vi "Next move 2.vi"(9 "Elevator states in":T1[](array[typedef])=[{"Elevator"={"Up Button"=FALSE, "Current floor"=1, "Down Button"=FALSE, "Car"={"Blank Button"=FALSE, "Blank Button 2"=FALSE, "Blank Button 3"=FALSE, "Blank Button 4"=FALSE, "Blank Button 5"=FALSE, "Blank Button 6"=FALSE, "Blank Button 7"=FALSE, "Blank Button 8"=FALSE, "Blank Button 9"=FALSE, "Blank Button 10"=FALSE, "Blank Button 11"=FALSE, "Blank Button 12"=FALSE, "Blank Button 13"=FALSE, "Blank Button 14"=FALSE, "Blank Button 15"=FALSE, "Blank Button 16"=FALSE, "Blank Button 17"=FALSE, "Blank Button 18"=FALSE, "Blank Button 19"=FALSE, "Blank Button 20"=FALSE}, "Close door"=FALSE}, "Destinations"=[], "Idle floor"=1, "Max floor"=7, "Min floor"=1, "Next floor"=0, "Move started"=timestamp(0 s since 1904-01-01), "Idle move"=FALSE}, {"Elevator"={"Up Button"=FALSE, "Current floor"=8, "Down Button"=FALSE, "Car"={"Blank Button"=FALSE, "Blank Button 2"=FALSE, "Blank Button 3"=FALSE, "Blank Button 4"=FALSE, "Blank Button 5"=FALSE, "Blank Button 6"=FALSE, "Blank Button 7"=FALSE, "Blank Button 8"=FALSE, "Blank Button 9"=FALSE, "Blank Button 10"=FALSE, "Blank Button 11"=FALSE, "Blank Button 12"=FALSE, "Blank Button 13"=FALSE, "Blank Button 14"=FALSE, "Blank Button 15"=FALSE, "Blank Button 16"=FALSE, "Blank Button 17"=FALSE, "Blank Button 18"=FALSE, "Blank Button 19"=FALSE, "Blank Button 20"=FALSE}, "Close door"=FALSE}, "Destinations"=[], "Idle floor"=8, "Max floor"=14, "Min floor"=8, "Next floor"=0, "Move started"=timestamp(0 s since 1904-01-01), "Idle move"=FALSE}, {"Elevator"={"Up Button"=FALSE, "Current floor"=1, "Down Button"=FALSE, "Car"={"Blank Button"=FALSE, "Blank Button 2"=FALSE, "Blank Button 3"=FALSE, "Blank Button 4"=FALSE, "Blank Button 5"=FALSE, "Blank Button 6"=FALSE, "Blank Button 7"=FALSE, "Blank Button 8"=FALSE, "Blank Button 9"=FALSE, "Blank Button 10"=FALSE, "Blank Button 11"=FALSE, "Blank Button 12"=FALSE, "Blank Button 13"=FALSE, "Blank Button 14"=FALSE, "Blank Button 15"=FALSE, "Blank Button 16"=FALSE, "Blank Button 17"=FALSE, "Blank Button 18"=FALSE, "Blank Button 19"=FALSE, "Blank Button 20"=FALSE}, "Close door"=FALSE}, "Destinations"=[], "Idle floor"=1, "Max floor"=14, "Min floor"=1, "Next floor"=0, "Move started"=timestamp(0 s since 1904-01-01), "Idle move"=FALSE}, {"Elevator"={"Up Button"=FALSE, "Current floor"=14, "Down Button"=FALSE, "Car"={"Blank Button"=FALSE, "Blank Button 2"=FALSE, "Blank Button 3"=FALSE, "Blank Button 4"=FALSE, "Blank Button 5"=FALSE, "Blank Button 6"=FALSE, "Blank Button 7"=FALSE, "Blank Button 8"=FALSE, "Blank Button 9"=FALSE, "Blank Button 10"=FALSE, "Blank Button 11"=FALSE, "Blank Button 12"=FALSE, "Blank Button 13"=FALSE, "Blank Button 14"=FALSE, "Blank Button 15"=FALSE, "Blank Button 16"=FALSE, "Blank Button 17"=FALSE, "Blank Button 18"=FALSE, "Blank Button 19"=FALSE, "Blank Button 20"=FALSE}, "Close door"=FALSE}, "Destinations"=[], "Idle floor"=14, "Max floor"=20, "Min floor"=6, "Next floor"=0, "Move started"=timestamp(0 s since 1904-01-01), "Idle move"=FALSE}]) -> (1 "Elevator states out":T1[](array[typedef])=[{"Elevator"={"Up Button"=FALSE, "Current floor"=1, "Down Button"=FALSE, "Car"={"Blank Button"=FALSE, "Blank Button 2"=FALSE, "Blank Button 3"=FALSE, "Blank Button 4"=FALSE, "Blank Button 5"=FALSE, "Blank Button 6"=FALSE, "Blank Button 7"=FALSE, "Blank Button 8"=FALSE, "Blank Button 9"=FALSE, "Blank Button 10"=FALSE, "Blank Button 11"=FALSE, "Blank Button 12"=FALSE, "Blank Button 13"=FALSE, "Blank Button 14"=FALSE, "Blank Button 15"=FALSE, "Blank Button 16"=FALSE, "Blank Button 17"=FALSE, "Blank Button 18"=FALSE, "Blank Button 19"=FALSE, "Blank Button 20"=FALSE}, "Close door"=FALSE}, "Destinations"=[], "Idle floor"=1, "Max floor"=7, "Min floor"=1, "Next floor"=0, "Move started"=timestamp(0 s since 1904-01-01), "Idle move"=FALSE}, {"Elevator"={"Up Button"=FALSE, "Current floor"=8, "Down Button"=FALSE, "Car"={"Blank Button"=FALSE, "Blank Button 2"=FALSE, "Blank Button 3"=FALSE, "Blank Button 4"=FALSE, "Blank Button 5"=FALSE, "Blank Button 6"=FALSE, "Blank Button 7"=FALSE, "Blank Button 8"=FALSE, "Blank Button 9"=FALSE, "Blank Button 10"=FALSE, "Blank Button 11"=FALSE, "Blank Button 12"=FALSE, "Blank Button 13"=FALSE, "Blank Button 14"=FALSE, "Blank Button 15"=FALSE, "Blank Button 16"=FALSE, "Blank Button 17"=FALSE, "Blank Button 18"=FALSE, "Blank Button 19"=FALSE, "Blank Button 20"=FALSE}, "Close door"=FALSE}, "Destinations"=[], "Idle floor"=8, "Max floor"=14, "Min floor"=8, "Next floor"=0, "Move started"=timestamp(0 s since 1904-01-01), "Idle move"=FALSE}, {"Elevator"={"Up Button"=FALSE, "Current floor"=1, "Down Button"=FALSE, "Car"={"Blank Button"=FALSE, "Blank Button 2"=FALSE, "Blank Button 3"=FALSE, "Blank Button 4"=FALSE, "Blank Button 5"=FALSE, "Blank Button 6"=FALSE, "Blank Button 7"=FALSE, "Blank Button 8"=FALSE, "Blank Button 9"=FALSE, "Blank Button 10"=FALSE, "Blank Button 11"=FALSE, "Blank Button 12"=FALSE, "Blank Button 13"=FALSE, "Blank Button 14"=FALSE, "Blank Button 15"=FALSE, "Blank Button 16"=FALSE, "Blank Button 17"=FALSE, "Blank Button 18"=FALSE, "Blank Button 19"=FALSE, "Blank Button 20"=FALSE}, "Close door"=FALSE}, "Destinations"=[], "Idle floor"=1, "Max floor"=14, "Min floor"=1, "Next floor"=0, "Move started"=timestamp(0 s since 1904-01-01), "Idle move"=FALSE}, {"Elevator"={"Up Button"=FALSE, "Current floor"=14, "Down Button"=FALSE, "Car"={"Blank Button"=FALSE, "Blank Button 2"=FALSE, "Blank Button 3"=FALSE, "Blank Button 4"=FALSE, "Blank Button 5"=FALSE, "Blank Button 6"=FALSE, "Blank Button 7"=FALSE, "Blank Button 8"=FALSE, "Blank Button 9"=FALSE, "Blank Button 10"=FALSE, "Blank Button 11"=FALSE, "Blank Button 12"=FALSE, "Blank Button 13"=FALSE, "Blank Button 14"=FALSE, "Blank Button 15"=FALSE, "Blank Button 16"=FALSE, "Blank Button 17"=FALSE, "Blank Button 18"=FALSE, "Blank Button 19"=FALSE, "Blank Button 20"=FALSE}, "Close door"=FALSE}, "Destinations"=[], "Idle floor"=14, "Max floor"=20, "Min floor"=6, "Next floor"=0, "Move started"=timestamp(0 s since 1904-01-01), "Idle move"=FALSE}], 2 "Served floors":u16[](array[numeric]), 5 "Served car":bool[](array[boolean]))   [LabVIEW 2019]
uses:
  Type defs/Elevator states.ctl
  Type defs/Elevator position.ctl
  Type defs/Car buttons.ctl
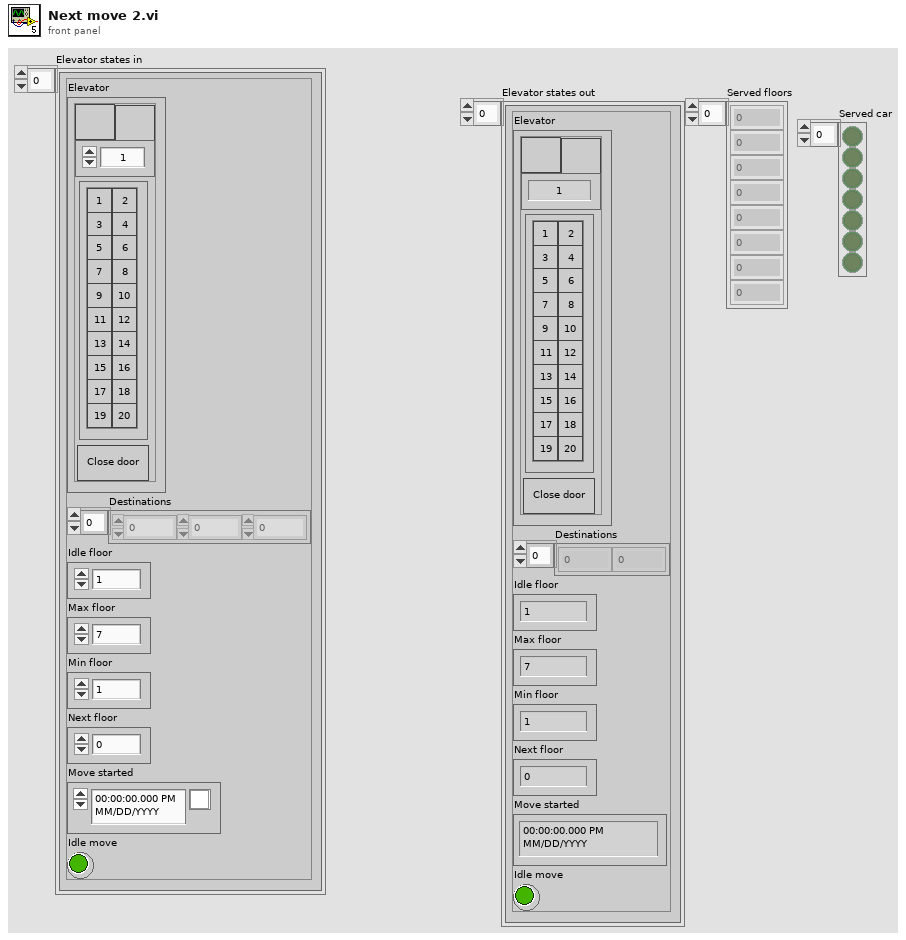
[diagram p1: front panel]
types:
  T1 = typedef "Elevator states.ctl" = cluster{"Elevator":T2, "Destinations":i32[], "Idle floor":u16, "Max floor":u16, "Min floor":u16, "Next floor":u16, "Move started":timestamp, "Idle move":bool}
  T2 = typedef "Elevator position.ctl" = cluster{"Up Button":bool, "Current floor":u16, "Down Button":bool, "Car":T3, "Close door":bool}
  T3 = typedef "Car buttons.ctl" = cluster{"Blank Button":bool, "Blank Button 2":bool, "Blank Button 3":bool, "Blank Button 4":bool, "Blank Button 5":bool, "Blank Button 6":bool, "Blank Button 7":bool, "Blank Button 8":bool, "Blank Button 9":bool, "Blank Button 10":bool, "Blank Button 11":bool, "Blank Button 12":bool, "Blank Button 13":bool, "Blank Button 14":bool, "Blank Button 15":bool, "Blank Button 16":bool, "Blank Button 17":bool, "Blank Button 18":bool, "Blank Button 19":bool, "Blank Button 20":bool}
  T4 = cluster{"Car[0]":bool, "Car[1]":bool, "Car[2]":bool, "Car[3]":bool, "Car[4]":bool, "Car[5]":bool, "Car[6]":bool, "Car[7]":bool, "Car[8]":bool, "Car[9]":bool, "Car[10]":bool, "Car[11]":bool, "Car[12]":bool, "Car[13]":bool, "Car[14]":bool, "Car[15]":bool, "Car[16]":bool, "Car[17]":bool, "Car[18]":bool, "Car[19]":bool}
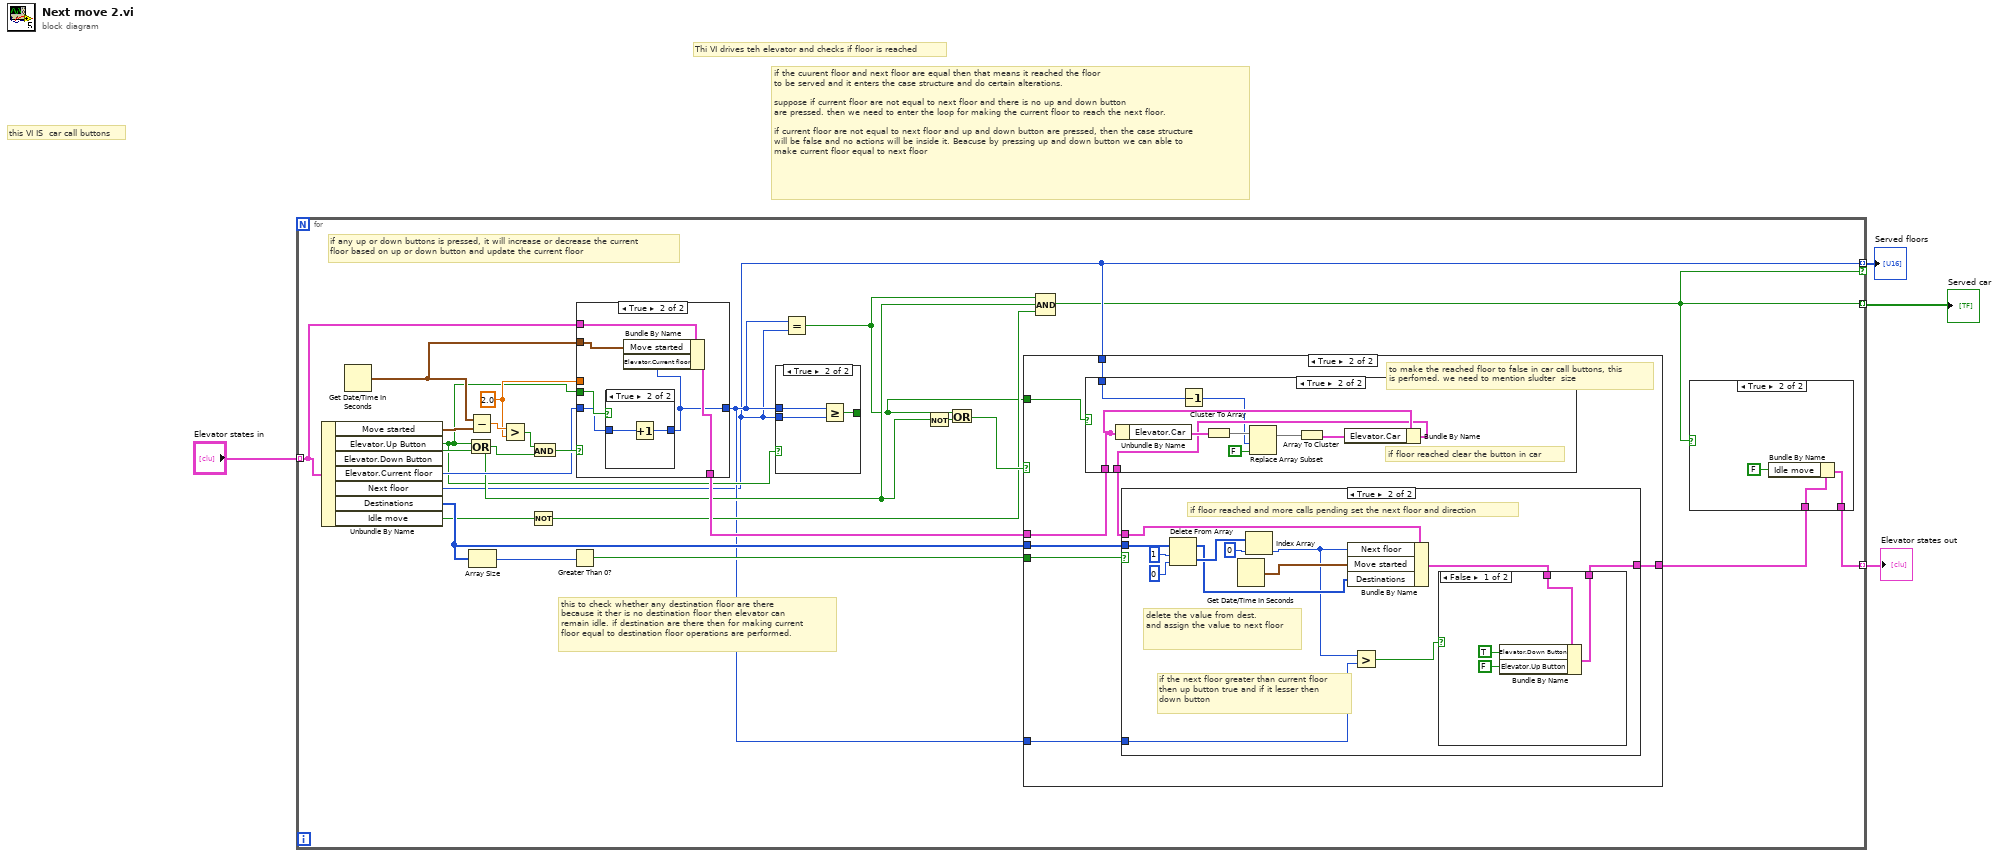
[diagram p0: block diagram]
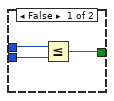
[diagram p2: hidden frame]
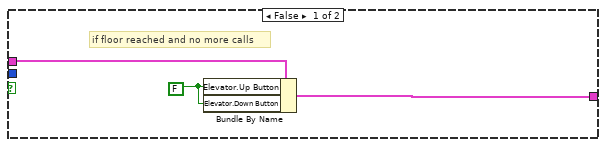
[diagram p5: hidden frame]
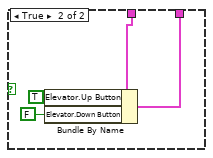
[diagram p6: hidden frame]
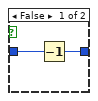
[diagram p9: hidden frame]
diagram:
  # "this VI IS  car call buttons"
  # "if the cuurent floor and next floor are equal then that means it reached the floor\nto be served and it enters the case structure and do certain alterations.\n\nsuppose if current floor are not equal to next floor and there is no up and down button \nare pressed. then we need to enter the loop for making the current floor to reach the next floor.\n\nif current floor are not equal to next floor and up and down button are pressed, then the case structure\nwill be false and no actions will be inside it. Beacuse by pressing up and down button we can able to\nmake current floor equal to next floor"
  # "Thi VI drives teh elevator and checks if floor is reached"
  n1 = for {
    tunnel: "Elevator states in" -> [w19] mode=indexing
    tunnel: [w11] -> w4 mode=indexing
    tunnel: [w7] -> w3 mode=indexing if=w5
    tunnel: [w5] -> w2 mode=indexing
    w24 = 2.0 ("y")
    # "this to check whether any destination floor are there\nbecause it ther is no destination floor then elevator can\nremain idle. if destination are there then for making current\nfloor equal to destination floor operations are performed."
    # "if any up or down buttons is pressed, it will increase or decrease the current\nfloor based on up or down button and update the current floor"
    n2 = Unbundle By Name(w19) -> ("Move started"=w25:timestamp, "Elevator.Up Button"=w9:bool, "Elevator.Down Button"=w29:bool, "Elevator.Current floor"=w18:u16, "Next floor"=w7:u16, "Destinations"=w21:i32[], "Idle move"=w14:bool)
    n3 = Get Date/Time In Seconds() -> (seconds since 1Jan1904=w10:timestamp)
    n4 = Or(x=w9, y=w29) -> (x .or. y?=w15:bool)
    n5 = Subtract(x=w10, y=w25) -> (x-y=w27:dbl)
    n6 = Array Size(array=w21) -> (size(s)=w23:i32)
    n7 = Greater?(x=w27, y=w24) -> (0:w26:bool)
    n8 = Not(x=w14) -> (.not. x?=w13:bool)
    n9 = And(x=w26, y=w15) -> (x .and. y?=w28:bool)
    n10 = Greater Than 0?(x=w23) -> (x > 0?=w22:bool)
    n11 = case shown="True" w28 {
      tunnel: w9 -> [_ w90]
      tunnel: w18 -> [w84 w89]
      tunnel: [w84 w86] -> w8
      tunnel: w19 -> [w83 w88]
      tunnel: w10 -> [_ w85]
      tunnel: w24 -> [_ _]
      tunnel: [w83 w87] -> w20
      frame False {
      }
      frame True {
        n12 = case shown="True" w90 {
          tunnel: w89 -> [w92 w94]
          tunnel: [w91 w93] -> w86
          frame False {
            n13 = Decrement(x=w92) -> (x-1=w91:u16)
          }
          frame True {
            n14 = Increment(x=w94) -> (x+1=w93:u16)
          }
        }
        n15 = Bundle By Name(cluster=w88, "Move started"=w85, "Elevator.Current floor"=w86) -> (w87:T1)
      }
    }
    n16 = case shown="True" w9 {
      tunnel: w8 -> [w32 w35]
      tunnel: w7 -> [w31 w34]
      tunnel: [w30 w33] -> _
      frame False {
        n17 = Less Or Equal?(x=w32, y=w31) -> (x <= y?=w30:bool)
      }
      frame True {
        n18 = Greater Or Equal?(x=w35, y=w34) -> (x >= y?=w33:bool)
      }
    }
    n19 = Equal?(x=w8, y=w7) -> (x = y?=w6:bool)
    n20 = Not(x=w15) -> (.not. x?=w16:bool)
    n21 = Or(x=w6, y=w16) -> (x .or. y?=w17:bool)
    n22 = case shown="True" w17 {
      tunnel: w22 -> [_ w48]
      tunnel: w21 -> [_ w47]
      tunnel: w20 -> [w40 w43]
      tunnel: [w40 w46] -> w12
      tunnel: w8 -> [_ w45]
      tunnel: w7 -> [_ w44]
      tunnel: w6 -> [_ w41]
      frame False {
        # "if floor not reached and elevator is moving"
      }
      frame True {
        # "to make the reached floor to false in car call buttons, this\nis perfomed. we need to mention sludter  size"
        n23 = case shown="True" w41 {
          tunnel: w44 -> [_ w79]
          tunnel: w43 -> [w73 w77]
          tunnel: [w73 w75] -> w42
          frame False {
          }
          frame True {
            # "if floor reached clear the button in car"
            n24 = Unbundle By Name(w77) -> ("Elevator.Car"=w82:T3)
            n25 = Decrement(x=w79) -> (x-1=w74:u16)
            n26 = Cluster To Array(cluster=w82) -> (array=w81:bool[])
            n27 = Replace Array Subset(array=w81, new element=FALSE ("new element/subarray"), index=w74) -> (w78:bool[])
            n28 = Array To Cluster(array=w78) -> (cluster=w76:T4)
            n29 = Bundle By Name(cluster=w77, "Elevator.Car"=w76) -> (w75:T1)
          }
        }
        n30 = case shown="True" w48 {
          tunnel: w47 -> [_ w64]
          tunnel: w42 -> [w51 w59]
          tunnel: [w49 w54] -> w46
          tunnel: w45 -> [_ w52]
          frame False {
            w50 = FALSE ("Elevator.Up Button")
            # "if floor reached and no more calls"
            n31 = Bundle By Name(cluster=w51, "Elevator.Up Button"=w50, "Elevator.Down Button"=w50) -> (w49:T1)
          }
          frame True {
            # "if the next floor greater than current floor\nthen up button true and if it lesser then \ndown button"
            # "delete the value from dest.\nand assign the value to next floor"
            # "if floor reached and more calls pending set the next floor and direction"
            n32 = Delete From Array(array=w64, length=1, index=0) -> (deleted portion=w61:i32[], array with subset deleted=w57:i32[])
            n33 = Get Date/Time In Seconds() -> (seconds since 1Jan1904=w58:timestamp)
            n34 = Index Array(array=w61, index=0) -> (element=w53:i32)
            n35 = Bundle By Name(cluster=w59, "Next floor"=w53, "Move started"=w58, "Destinations"=w57) -> (w55:T1)
            n36 = Greater?(x=w53, y=w52) -> (0:w56:bool)
            n37 = case shown="False" w56 {
              tunnel: w55 -> [w68 w72]
              tunnel: [w67 w70] -> w54
              frame False {
                n38 = Bundle By Name(cluster=w68, "Elevator.Down Button"=TRUE, "Elevator.Up Button"=FALSE) -> (w67:T1)
              }
              frame True {
                n39 = Bundle By Name(cluster=w72, "Elevator.Up Button"=TRUE, "Elevator.Down Button"=FALSE) -> (w70:T1)
              }
            }
          }
        }
      }
    }
    n40 = Compound Arithmetic op=AND(w6, w15, w13) -> (w5:bool)
    n41 = case shown="True" w5 {
      tunnel: w12 -> [w36 w39]
      tunnel: [w36 w37] -> w11
      frame False {
      }
      frame True {
        n42 = Bundle By Name(cluster=w39, "Idle move"=FALSE) -> (w37:T1)
      }
    }
  }
  "Elevator states out" <- w4
  "Served floors" <- w3
  "Served car" <- w2
